vi "CreateBeamLineTotalSourceIonEnergyNode.vi"(8 "Error In":errorcluster, 10 "Beam Line":T1={"Type"=enum."Ion Beam Analysis", "Ion"=enum."H", "Charge State"=0, "Total Source Ion Energy (kV)"=nan} {"Charge State" min=1}, 11 "DOM Document In":refnum<k20>) -> (0 "Error out":errorcluster, 2 "Beam Line Total Source Ion Energy Node":refnum<k20>, 3 "DOM Document Out":refnum<k20>)   [LabVIEW 2012]
uses:
  BeamLine.ctl
  BeamLineType.ctl
  BeamLineIon.ctl
  <resource>/objmgr/DOMUserDefRef.rc
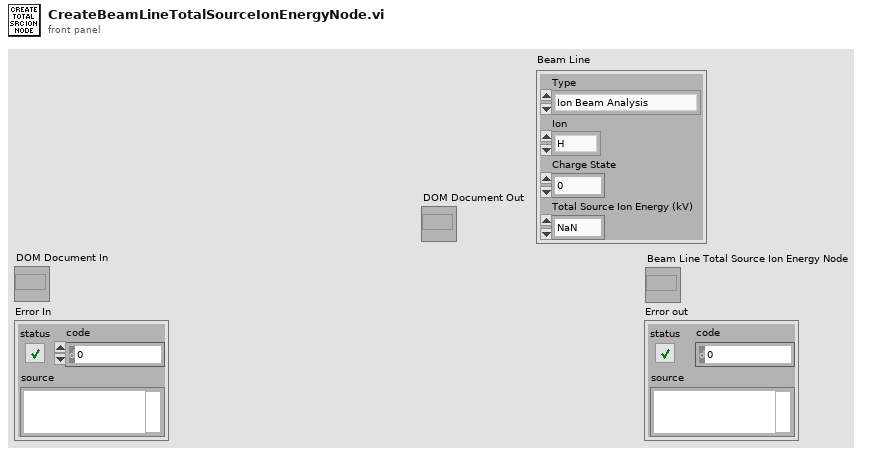
[diagram p1: front panel]
types:
  T1 = typedef "BeamLine.ctl" = cluster{"Type":T2, "Ion":T3, "Charge State":u8, "Total Source Ion Energy (kV)":dbl}
  T2 = typedef "BeamLineType.ctl" = enum16{"Ion Beam Analysis", "Auxiliary", "Radiation Damage"}
  T3 = typedef "BeamLineIon.ctl" = enum16{"H", "He", "C", "Fe", "Ni", "Pt", "Si", "Ag", "Au"}
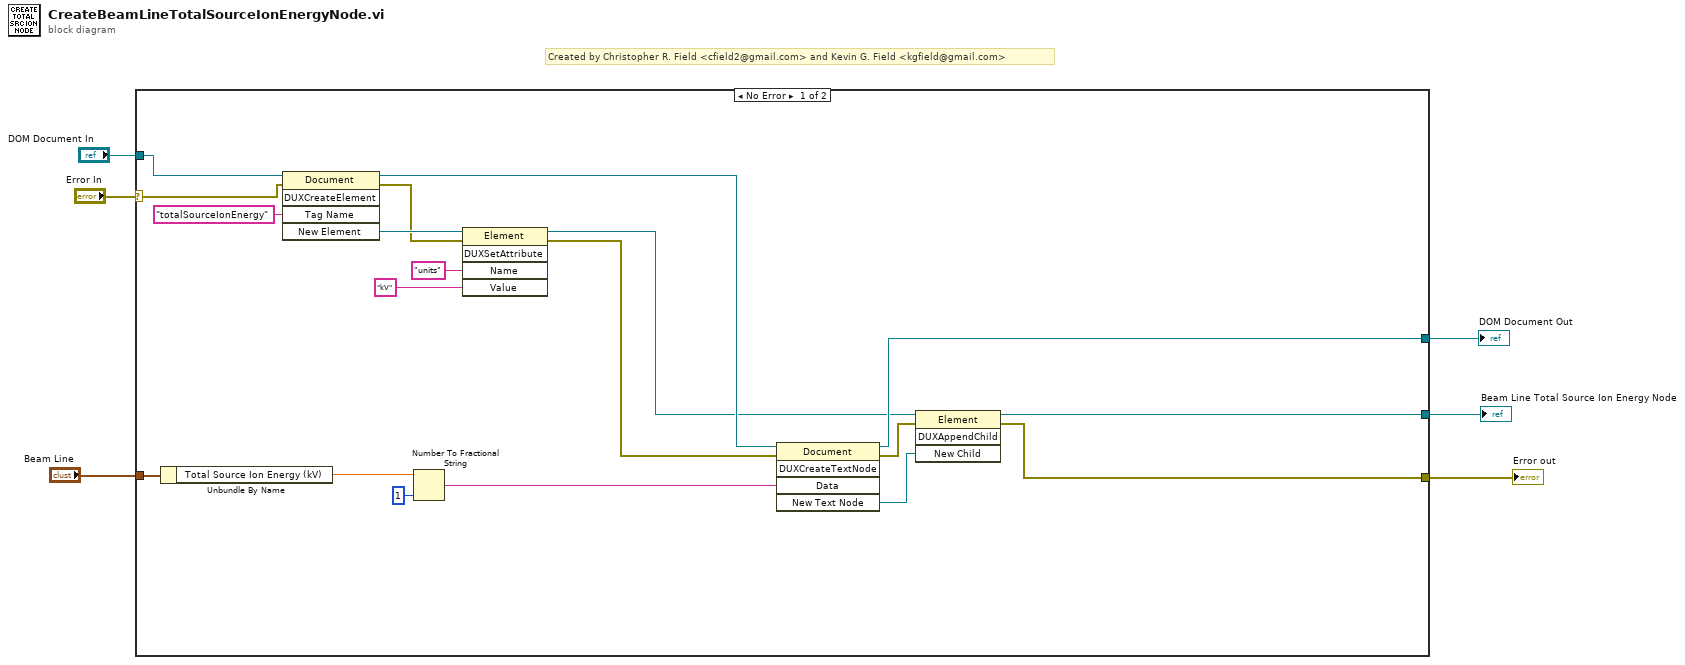
[diagram p0: block diagram]
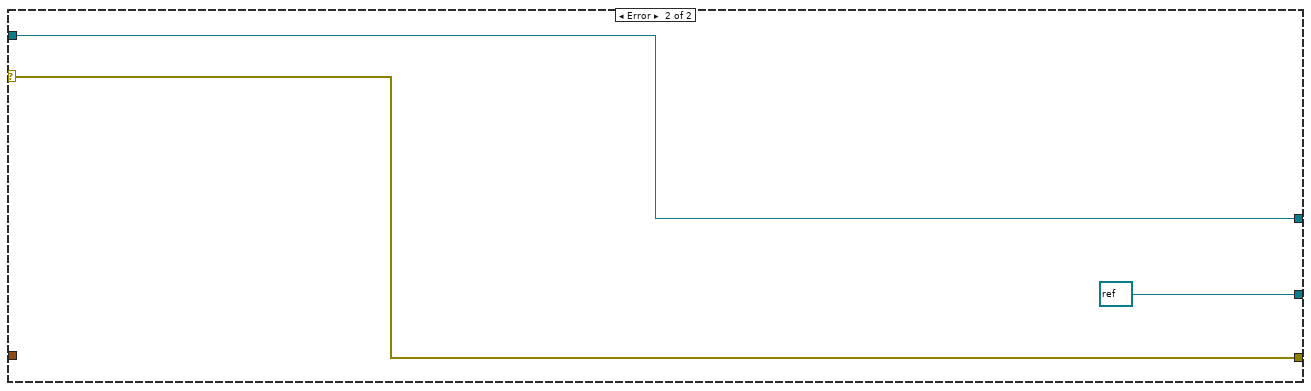
[diagram p2: hidden frame]
diagram:
  # "Created by Christopher R. Field <cfield2@gmail.com> and Kevin G. Field <kgfield@gmail.com>"
  n1 = case shown="No Error" "Error In" {
    selector: "Error In" -> [w18 w27]
    tunnel: "DOM Document In" -> [w25 w28]
    tunnel: [w24 refnum<k20> refnum ("Operator Node 2")] -> w5
    tunnel: [w23 w27] -> w4
    tunnel: "Beam Line" -> [w19 _]
    tunnel: [w17 w28] -> w2
    frame No Error {
      n2 = Unbundle By Name(w19) -> ("Total Source Ion Energy (kV)"=w15:dbl)
      n3 = invoke class="Document" method="DUXCreateElement"(reference=w25, error in=w18, "Tag Name"="totalSourceIonEnergy") -> (reference out=w16:refnum<k20>, error out=w9:errorcluster, "New Element"=w11:refnum<k20>)  [unwired: 2 in, 2 out]
      n4 = Number To Fractional String(number=w15, precision (6)=i16 1) -> (F-format string=w13:string)  [unwired: 2 in]
      n5 = invoke class="Element" method="DUXSetAttribute"(reference=w11, error in=w9, "Name"="units", "Value"="kV" ("Attribute Value")) -> (reference out=w7:refnum<k20>, error out=w8:errorcluster)  [unwired: 1 in, 3 out]
      n6 = invoke class="Document" method="DUXCreateTextNode"(reference=w16, error in=w8, "Data"=w13) -> (reference out=w17:refnum<k20>, error out=w21:errorcluster, "New Text Node"=w20:refnum<k20>)  [unwired: 2 in, 2 out]
      n7 = invoke class="Element" method="DUXAppendChild"(reference=w7, error in=w21, "New Child"=w20) -> (reference out=w24:refnum<k20>, error out=w23:errorcluster)  [unwired: 1 in, 2 out]
    }
    frame Error {
    }
  }
  "Beam Line Total Source Ion Energy Node" <- w5
  "Error out" <- w4
  "DOM Document Out" <- w2
